vi "Location Map View.vi"() -> ()   [LabVIEW 2012]
panel:
  in  "stop":bool
  out "XY Graph":cluster{dbl[], dbl[]}(graph)
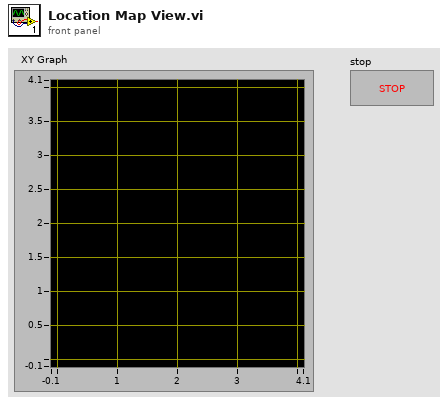
[diagram p1: front panel]
types:
  T1 = cluster{"Width":u16, "Style":enum32{"Solid", "Dash", "Dot", "DashDot", "DashDotDot"}}
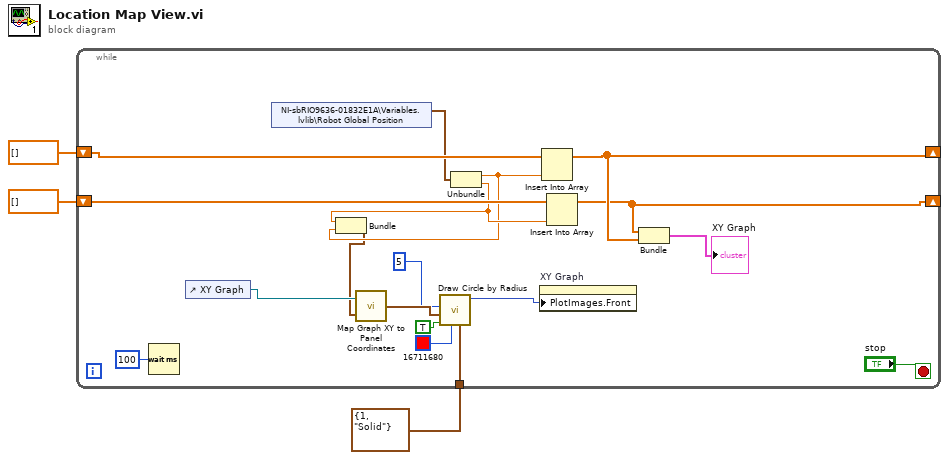
[diagram p0: block diagram]
diagram:
  n1 = while {
    shift-right: [w18] -> _
    shift-left: dbl[] [] -> [w19]
    shift-right: [w20] -> _
    shift-left: dbl[] [] -> [w21]
    tunnel: T1 {"Width"=1, "Style"=enum."Solid"} ("pen") -> [w11]
    stop <- "stop" stop-if-true
    n2 = Wait (ms)(milliseconds to wait=u32 100) -> ()  [unwired: 1 out]
    n3 = control-ref of="XY Graph"() -> (w9:refnum<vi>)
    n4 = shared-variable "NI-sbRIO9636-01832E1A\\Variables.lvlib\\Robot Global Position"() -> (w13:cluster{"Global X":dbl, "Global Y":dbl})  [unwired: 1 in, 1 out]
    n5 = Unbundle(w13) -> ("Global X"=w5:dbl, "Global Y"=w6:dbl)
    n6 = Bundle("Global Y"=w6, "Global X"=w5) -> (w4:cluster{"Global Y":dbl, "Global X":dbl})  [unwired: 1 in]
    n7 = call "Map Graph XY to Panel Coordinates.vi"("XY"=w4, "Graph"=w9) -> ("Coords"=w14:cluster{i32, i32})
    n8 = call <vilib>:"Draw Circle by Radius.vi"("pen"=w11, "color(black)"=u32 16711680, "fill?(F)"=TRUE, "pixel center"=w14, "radius"=i16 5) -> ("new picture"=w12:picture)  [unwired: 6 in]
    n9 = property on="XY Graph" class="XYGraph (strict)"("PlotImages.Front"=w12) -> ()  [unwired: 2 in, 2 out]
    n10 = Insert Into Array(array=w21, new element=w5) -> (w20:dbl[])  [unwired: 1 in]
    n11 = Insert Into Array(array=w19, new element=w6) -> (w18:dbl[])  [unwired: 1 in]
    n12 = Bundle(w18, w20) -> (→"XY Graph":cluster{dbl[], dbl[]})  [unwired: 1 in]
  }
